vi "PowNon.vi"(8 "error in":errorcluster, 9 "Type":u16(ring) items=["LAST+OFF", "LAST", "RESET"], 11 "VISA resource name":refnum<visa-resource-name>) -> (0 "error out":errorcluster, 3 "VISA resource name out":refnum<visa-resource-name>)   [LabVIEW 2015, in "IT-M7700.lvlib"]
doc: "This command is used to set the display and output status of some parameter default values when the power supply is powered on.\n<b>Type</b>\n0: LAST+OFF\n1: LAST\n2: RESET"
uses:
  <instrlib>/IT-M7700/IT-M7700.lvlib
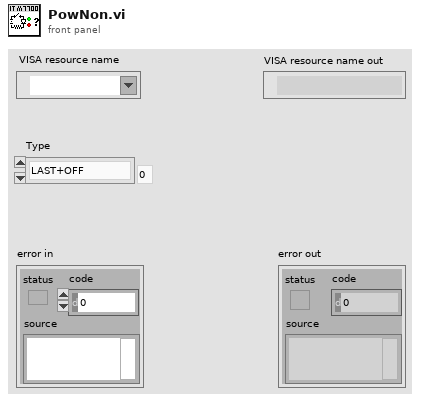
[diagram p1: front panel]
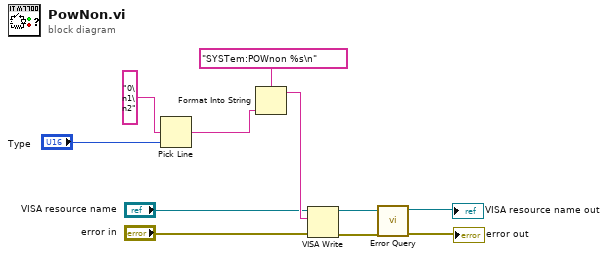
[diagram p0: block diagram]
diagram:
  n1 = Pick Line(multi-line string="0\n1\n2", line index="Type") -> (output string=w6:string)  [unwired: 1 in]
  n2 = Format Into String(format string="SYSTem:POWnon %s\n", w6) -> (resulting string=w9:string)  [unwired: 2 in, 1 out]
  n3 = VISA Write(VISA resource name="VISA resource name", write buffer=w9, error in (no error)="error in") -> (VISA resource name out=w5:refnum<visa-resource-name>, error out=w4:errorcluster)  [unwired: 1 out]
  n4 = call <instrlib>:"Error Query.vi"("error in"=w4, "VISA resource name"=w5) -> ("error out"=→"error out":errorcluster, "VISA resource name out"=→"VISA resource name out":refnum<visa-resource-name>)  [unwired: 6 in, 2 out]
